vi "Read Limit Switch Status.vi"(0 "class data in":refnum<class "MB_ENGINE.lvclass">, 11 "error in (no error)":errorcluster) -> (4 "class data out":refnum<class "MB_ENGINE.lvclass">, 6 "Limits":T1, 15 "error out":errorcluster)   [LabVIEW 2019, in "MB_ENGINE.lvclass"]
uses:
  MB_ENGINE.lvclass
  Limits Status.ctl
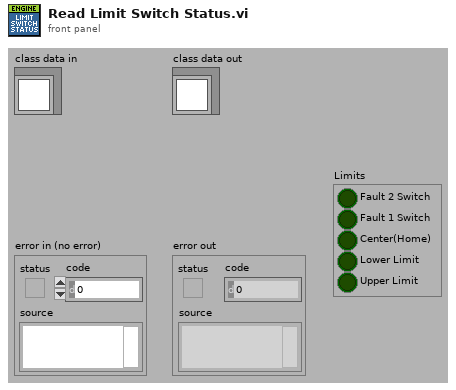
[diagram p1: front panel]
types:
  T1 = typedef "MB_ENGINE.lvclass/Limits Status.ctl" = cluster{"Fault 2 Switch":bool, "Fault 1 Switch":bool, "Center(Home)":bool, "Lower Limit":bool, "Upper Limit":bool}
  T2 = cluster{"Boolean array[0]":bool, "Boolean array[1]":bool, "Boolean array[2]":bool, "Boolean array[3]":bool, "Boolean array[4]":bool}
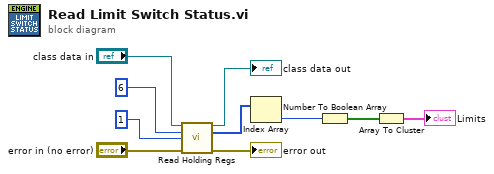
[diagram p0: block diagram]
diagram:
  n1 = call-dynamic "Read Holding Regs.vi"("reference in"="class data in", "starting address"=u16 6, "number of inputs"=u16 1, "error in (no error)"="error in (no error)") -> ("reference out"=→"class data out":refnum<class "MB_ENGINE.lvclass">, "register values"=w2:u16[], "error out"=→"error out":errorcluster)  [unwired: 9 in]
  n2 = Index Array(array=w2) -> (element=w5:u16)  [unwired: 1 in]
  n3 = Number To Boolean Array(number=w5) -> (Boolean array=w4:bool[])
  n4 = Array To Cluster(array=w4) -> (cluster=→"Limits":T2)
